vi "ATR.vi"() -> ()   [LabVIEW 2017]
panel:
  out "ArrAHU":string[][](array[string])
  out "ArrEbay":string[][](array[string])
  out "Mort Temp":string[][](array[string])
  out "Aux":string[][](array[string])
  out "Burnin":string[][](array[string])
  out "Temp Algo":string[][](array[string])
  out "Speed":string[][](array[string])
  out "Tempreature calibration":string[][](array[string])
  out "StopTime":string[][](array[string])
  out "Enable":string[][](array[string])
  out "Communication":string[][](array[string])
  out "Visual Inspection":string[][](array[string])
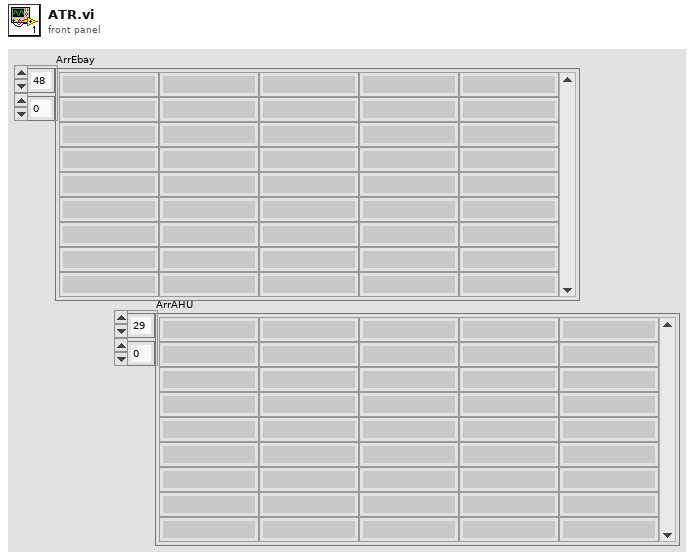
[diagram p1: front panel]
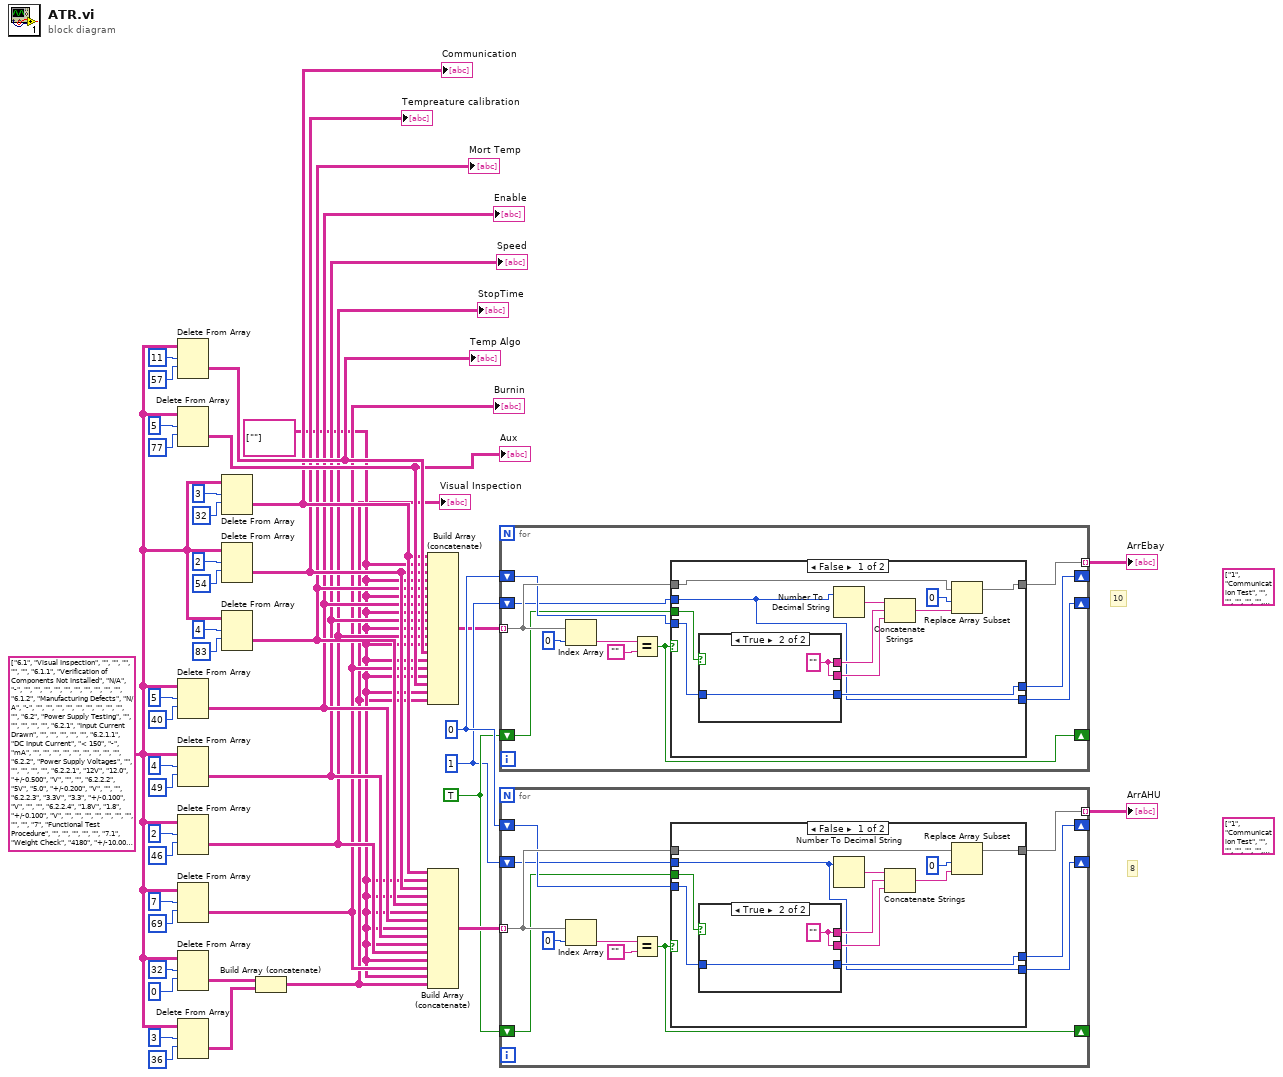
[diagram p0: block diagram]
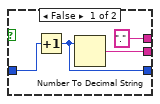
[diagram p2: hidden frame]
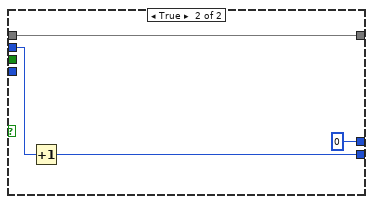
[diagram p3: hidden frame]
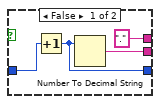
[diagram p4: hidden frame]
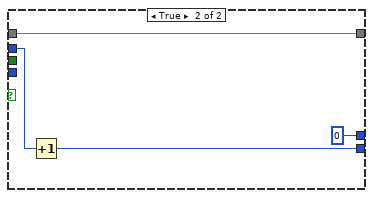
[diagram p5: hidden frame]
diagram:
  (unwired) string[][] [["1", "Communication Test", "", "", "", "", ""], ["1.1", "Serial RS-232", "N/A", "-", "", "", ""], ["1.2", "CAN Bus", "N/A", "-", "", "", ""], ["", "", "", "", "", "", ""], ["2", "Temperature Sensor Calibration Test", "", "", "", "", ""], ["2.1", "Sensor Reading Analog Offset", "0", "+/-0.100", ".", "", ""], ["", "", "", "", "", "", ""], ["3", "Motor Temp. Test", "", "", "", "", ""], ["3.1", "60 Degree", "60", "+/-3.00", "C", "", ""], ["3.2", "90 Degree", "90", "+/-3.00", "C", "", ""], ["3.3", "120 Degree", "120", "+/-3.00", "C", "", ""], ["", "", "", "", "", "", ""], ["4", "Enable Test", "", "", "", "", ""], ["4.1", "Fan Speed at Opened Enable ", "5000", "+/-200.0", "rpm", "", ""], ["4.2", "Fan Speed at Opened Enable ", "0", "+/-200.0", "rpm", "", ""], ["4.3", "Fan Speed at Closed Enable ", "5000", "+/-200.0", "rpm", "", ""], ["4.4", "Motor Rotation Direction", "Counter-clockwise (Inlet)", "-", "", "", ""], ["", "", "", "", "", "", ""], ["5", "Speed Command Test", "", "", "", "", ""], ["5.1", "Fan Speed", "6000", "+/-200.0", "rpm", "", ""], ["5.2", "Fan Speed", "11500", "+/-200.0", "rpm", "", ""], ["5.3", "Fan Speed", "15100", "+/-200.0", "rpm", "", ""], ["", "", "", "", "", "", ""], ["6", "Stop Time Test ", "", "", "", "", ""], ["6.1", "Motor Stop time", "< 50", "-", "sec", "", ""], ["", "", "", "", "", "", ""], ["7", "Burn-in Test", "", "", "", "", ""], ["7.1", "DC Input Current", "50", "+/-5.000", "A", "", ""], ["7.2", "Fan Speed", "15100", "+/-200.0", "rpm", "", ""], ["7.3", "Ambient Temperature", "25", "+/-13.00", "C", "", ""], ["7.4", "After 10 min of operation", "", "-", "C", "", ""], ["7.5", "After 20 min of operation", "", "-", "C", "", ""], ["7.6", "After 30 min of operation", "", "-", "C", "", ""], ["", "", "", "", "", "", ""], ["8", "Visual Inspection", "", "", "", "", ""], ["8.1", "Verification of Components Not Installed", "N/A", "-", "", "", ""], ["", "", "", "", "", "", ""], ["9", "Manufacturing Defects", "N/A", "-", "", "", ""], ["", "", "", "", "", "", ""], ["10", "Power Supply Testing", "", "", "", "", ""], ["10.1", "Input Current Drawn", "", "", "", "", ""], ["10.2", "DC Input Current", "< 150", "-", "mA", "", ""], ["", "", "", "", "", "", ""], ["11", "Power Supply Voltages", "", "", "", "", ""], ["11.1", "12V", "12.0", "+/-0.500", "V", "", ""], ["11.2", "5V", "5.0", "+/-0.200", "V", "", ""], ["11.3", "3.3V", "3.3", "+/-0.100", "V", "", ""], ["11.4", "1.8V", "1.8", "+/-0.100", "V", "", ""], ["", "", "", "", "", "", ""], ["12", "Functional Test Procedure", "", "", "", "", ""], ["12.1", "Weight Check", "4180", "+/-10.00", "gr", "", ""], ["", "", "", "", "", "", ""], ["13", "Insulation Resistance Test", "", "", "", "", ""], ["13.1", "J3.B to Chassis", "> 1M", "-", "W", "", ""], ["13.2", "J1.16 to Chassis", "> 100K", "-", "W", "", ""], ["", "", "", "", "", "", ""], ["14", "Bonding Resistance", "", "", "", "", ""], ["14.1", "J1 Body to Chassis", "< 2m", "-", "W", "", ""], ["14.2", "J2  Body to Chassis", "< 2m", "-", "W", "", ""], ["14.3", "J3  Body to Chassis", "< 2m", "-", "W", "", ""], ["", "", "", "", "", "", ""], ["15", "CANbus Resistance Test", "", "", "", "", ""], ["15.1", "J1.17 to J1.18", "> 10K", "-", "W", "", ""], ["", "", "", "", "", "", ""], ["16", "Sealing Test", "N/A", "-", "", "", ""], ["", "", "", "", "", "", ""], ["17", "Performances Tests", "", "", "", "", ""], ["17.1", "Reverse Polarity Test", "", "", "", "", ""], ["17.2", "DC Input Current", "< 1", "-", "mA", "", ""]] ("ArrAHU 2")
  (unwired) string[][] [["1", "Communication Test", "", "", "", "", ""], ["1.1", "Serial RS-232", "N/A", "-", "", "", ""], ["1.2", "CAN Bus", "N/A", "-", "", "", ""], ["", "", "", "", "", "", ""], ["2", "Temperature Sensor Calibration Test", "", "", "", "", ""], ["2.1", "Sensor Reading Analog Offset", "0", "+/-0.100", ".", "", ""], ["", "", "", "", "", "", ""], ["3", "Motor Temp. Test", "", "", "", "", ""], ["3.1", "60 Degree", "60", "+/-3.00", "C", "", ""], ["3.2", "90 Degree", "90", "+/-3.00", "C", "", ""], ["3.3", "120 Degree", "120", "+/-3.00", "C", "", ""], ["", "", "", "", "", "", ""], ["4", "Enable Test", "", "", "", "", ""], ["4.1", "Fan Speed at Opened Enable ", "5000", "+/-200.0", "rpm", "", ""], ["4.2", "Fan Speed at Opened Enable ", "0", "+/-200.0", "rpm", "", ""], ["4.3", "Fan Speed at Closed Enable ", "5000", "+/-200.0", "rpm", "", ""], ["4.4", "Motor Rotation Direction", "Counter-clockwise (Inlet)", "-", "", "", ""], ["", "", "", "", "", "", ""], ["5", "Speed Command Test", "", "", "", "", ""], ["5.1", "Fan Speed", "6000", "+/-200.0", "rpm", "", ""], ["5.2", "Fan Speed", "11500", "+/-200.0", "rpm", "", ""], ["5.3", "Fan Speed", "15100", "+/-200.0", "rpm", "", ""], ["", "", "", "", "", "", ""], ["6", "Stop Time Test ", "", "", "", "", ""], ["6.1", "Motor Stop time", "< 50", "-", "sec", "", ""], ["", "", "", "", "", "", ""], ["7", "Temperature Control Algorithm Test", "", "", "", "", ""], ["7.1", "Tair <   68 ± 2 oC", "6000", "+/-200.0", "rpm", "", ""], ["7.2", "Measured Temp.", "", "", "C", "", ""], ["7.3", "Tair >= 68 ± 2 oC", "11500", "+/-200.0", "rpm", "", ""], ["7.4", "Transition Temp.", "", "", "C", "", ""], ["7.5", "Tair >= 88 ± 2 oC", "15100", "+/-400.0", "rpm", "", ""], ["7.6", "Transition Temp.", "", "", "C", "", ""], ["7.7", "Tair <= 80 ± 2 oC", "11500", "+/-200.0", "rpm", "", ""], ["7.8", "Transition Temp.", "", "", "C", "", ""], ["7.9", "Tair <= 60 ± 2 oC", "6000", "+/-200.0", "rpm", "", ""], ["7.10", "Transition Temp.", "", "", "C", "", ""], ["", "", "", "", "", "", ""], ["8", "Burn-in Test", "", "", "", "", ""], ["8.1", "DC Input Current", "50", "+/-5.000", "A", "", ""], ["8.2", "Fan Speed", "15100", "+/-200.0", "rpm", "", ""], ["8.3", "Ambient Temperature", "25", "+/-13.00", "C", "", ""], ["8.4", "After 10 min of operation", "", "-", "C", "", ""], ["8.5", "After 20 min of operation", "", "-", "C", "", ""], ["8.6", "After 30 min of operation", "", "-", "C", "", ""], ["", "", "", "", "", "", ""], ["9", "Auxiliary", "", "", "", "", ""], ["9.1", "Auxiliary Cooling Fan ON", "60", "+/-2.00", "C", "", ""], ["9.2", "Fan status", "ON", "-", "-", "", ""], ["9.3", "Auxiliary Cooling Fan OFF", "55", "+/-2.00", "C", "", ""], ["9.4", "Fan status", "OFF", "-", "-", "", ""], ["", "", "", "", "", "", ""], ["10", "Visual Inspection", "", "", "", "", ""], ["10.1", "Verification of Components Not Installed", "N/A", "-", "", "", ""], ["", "", "", "", "", "", ""], ["11", "Manufacturing Defects", "N/A", "-", "", "", ""], ["", "", "", "", "", "", ""], ["12", "Power Supply Testing", "", "", "", "", ""], ["12.1", "Input Current Drawn", "", "", "", "", ""], ["12.2", "DC Input Current", "< 150", "-", "mA", "", ""], ["", "", "", "", "", "", ""], ["13", "Power Supply Voltages", "", "", "", "", ""], ["13.1", "12V", "12.0", "+/-0.500", "V", "", ""], ["13.2", "5V", "5.0", "+/-0.200", "V", "", ""], ["13.3", "3.3V", "3.3", "+/-0.100", "V", "", ""], ["13.4", "1.8V", "1.8", "+/-0.100", "V", "", ""], ["", "", "", "", "", "", ""], ["14", "Functional Test Procedure", "", "", "", "", ""], ["14.1", "Weight Check", "4180", "+/-10.00", "gr", "", ""], ["", "", "", "", "", "", ""], ["15", "Insulation Resistance Test", "", "", "", "", ""], ["15.1", "J3.B to Chassis", "> 1M", "-", "W", "", ""], ["15.2", "J1.16 to Chassis", "> 100K", "-", "W", "", ""], ["", "", "", "", "", "", ""], ["16", "Bonding Resistance", "", "", "", "", ""], ["16.1", "J1 Body to Chassis", "< 2m", "-", "W", "", ""], ["16.2", "J2  Body to Chassis", "< 2m", "-", "W", "", ""], ["16.3", "J3  Body to Chassis", "< 2m", "-", "W", "", ""], ["", "", "", "", "", "", ""], ["17", "CANbus Resistance Test", "", "", "", "", ""], ["17.1", "J1.17 to J1.18", "> 10K", "-", "W", "", ""], ["", "", "", "", "", "", ""], ["18", "Sealing Test", "N/A", "-", "", "", ""], ["", "", "", "", "", "", ""], ["19", "Performances Tests", "", "", "", "", ""], ["19.1", "Reverse Polarity Test", "", "", "", "", ""], ["19.2", "DC Input Current", "< 1", "-", "mA", "", ""]] ("ArrEbay 2")
  w8 = string[][] [[""]] ("array")
  w4 = TRUE
  w3 = 1
  w5 = 0
  w19 = string[][] [["6.1", "Visual Inspection", "", "", "", "", ""], ["6.1.1", "Verification of Components Not Installed", "N/A", "-", "", "", ""], ["", "", "", "", "", "", ""], ["6.1.2", "Manufacturing Defects", "N/A", "-", "", "", ""], ["", "", "", "", "", "", ""], ["6.2", "Power Supply Testing", "", "", "", "", ""], ["6.2.1", "Input Current Drawn", "", "", "", "", ""], ["6.2.1.1", "DC Input Current", "< 150", "-", "mA", "", ""], ["", "", "", "", "", "", ""], ["6.2.2", "Power Supply Voltages", "", "", "", "", ""], ["6.2.2.1", "12V", "12.0", "+/-0.500", "V", "", ""], ["6.2.2.2", "5V", "5.0", "+/-0.200", "V", "", ""], ["6.2.2.3", "3.3V", "3.3", "+/-0.100", "V", "", ""], ["6.2.2.4", "1.8V", "1.8", "+/-0.100", "V", "", ""], ["", "", "", "", "", "", ""], ["7", "Functional Test Procedure", "", "", "", "", ""], ["7.1", "Weight Check", "4180", "+/-10.00", "gr", "", ""], ["", "", "", "", "", "", ""], ["7.2", "Insulation Resistance Test", "", "", "", "", ""], ["7.2.1", "J3.B to Chassis", "> 1M", "-", "W", "", ""], ["7.2.2", "J1.16 to Chassis", "> 100K", "-", "W", "", ""], ["", "", "", "", "", "", ""], ["7.2", "Bonding Resistance", "", "", "", "", ""], ["7.2.3", "J1 Body to Chassis", "< 2m", "-", "W", "", ""], ["7.2.4", "J2  Body to Chassis", "< 2m", "-", "W", "", ""], ["7.2.5", "J3  Body to Chassis", "< 2m", "-", "W", "", ""], ["", "", "", "", "", "", ""], ["7.2.1", "CANbus Resistance Test", "", "", "", "", ""], ["7.2.1.1", "J1.17 to J1.18", "> 10K", "-", "W", "", ""], ["", "", "", "", "", "", ""], ["7.3", "Sealing Test", "N/A", "-", "", "", ""], ["", "", "", "", "", "", ""], ["7.4", "Communication Test", "", "", "", "", ""], ["7.4.1", "Serial RS-232", "N/A", "-", "", "", ""], ["7.4.2", "CAN Bus", "N/A", "-", "", "", ""], ["", "", "", "", "", "", ""], ["7.5", "Performances Tests", "", "", "", "", ""], ["7.5.1", "Reverse Polarity Test", "", "", "", "", ""], ["7.5.1.1", "DC Input Current", "< 1", "-", "mA", "", ""], ["", "", "", "", "", "", ""], ["7.5.2", "Enable Test", "", "", "", "", ""], ["7.5.2.1", "Fan Speed at Opened Enable ", "5000", "+/-200.0", "rpm", "", ""], ["7.5.2.2", "Fan Speed at Opened Enable ", "0", "+/-200.0", "rpm", "", ""], ["7.5.2.3", "Fan Speed at Closed Enable ", "5000", "+/-200.0", "rpm", "", ""], ["7.5.2.4", "Motor Rotation Direction", "Counter-clockwise (Inlet)", "-", "", "", ""], ["", "", "", "", "", "", ""], ["7.5.3", "Stop Time Test ", "", "", "", "", ""], ["7.5.3.1", "Motor Stop time", "< 50", "-", "sec", "", ""], ["", "", "", "", "", "", ""], ["7.5.4", "Speed Command Test", "", "", "", "", ""], ["7.5.4.1", "Fan Speed", "6000", "+/-200.0", "rpm", "", ""], ["7.5.4.2", "Fan Speed", "11500", "+/-200.0", "rpm", "", ""], ["7.5.4.3", "Fan Speed", "15100", "+/-200.0", "rpm", "", ""], ["", "", "", "", "", "", ""], ["7.5.5", "Temperature Sensor Calibration Test", "", "", "", "", ""], ["7.5.5.1", "Sensor Reading Analog Offset", "0", "+/-0.100", ".", "", ""], ["", "", "", "", "", "", ""], ["7.5.6", "Temperature Control Algorithm Test", "", "", "", "", ""], ["7.5.6.1", "Tair <   68 ± 2 oC", "6000", "+/-200.0", "rpm", "", ""], ["7.5.6.2", "Measured Temp.", "", "", "C", "", ""], ["7.5.6.3", "Tair >= 68 ± 2 oC", "11500", "+/-200.0", "rpm", "", ""], ["7.5.6.4", "Transition Temp.", "", "", "C", "", ""], ["7.5.6.5", "Tair >= 88 ± 2 oC", "15100", "+/-400.0", "rpm", "", ""], ["7.5.6.6", "Transition Temp.", "", "", "C", "", ""], ["7.5.6.7", "Tair <= 80 ± 2 oC", "11500", "+/-200.0", "rpm", "", ""], ["7.5.6.8", "Transition Temp.", "", "", "C", "", ""], ["7.5.6.9", "Tair <= 60 ± 2 oC", "6000", "+/-200.0", "rpm", "", ""], ["7.5.6.10", "Transition Temp.", "", "", "C", "", ""], ["", "", "", "", "", "", ""], ["7.5.7", "Burn-in Test", "", "", "", "", ""], ["7.5.7.1", "DC Input Current", "50", "+/-5.000", "A", "", ""], ["7.5.7.2", "Fan Speed", "15100", "+/-200.0", "rpm", "", ""], ["7.5.7.3", "Ambient Temperature", "25", "+/-13.00", "C", "", ""], ["7.5.7.4", "After 10 min of operation", "", "-", "C", "", ""], ["7.5.7.5", "After 20 min of operation", "", "-", "C", "", ""], ["7.5.7.6", "After 30 min of operation", "", "-", "C", "", ""], ["", "", "", "", "", "", ""], ["8", "Auxiliary", "", "", "", "", ""], ["8.1", "Auxiliary Cooling Fan ON", "60", "+/-2.00", "C", "", ""], ["8.2", "Fan status", "ON", "-", "-", "", ""], ["8.3", "Auxiliary Cooling Fan OFF", "55", "+/-2.00", "C", "", ""], ["8.4", "Fan status", "OFF", "-", "-", "", ""], ["", "", "", "", "", "", ""], ["9", "Motor Temp. Test", "", "", "", "", ""], ["9.1", "60 Degree", "60", "+/-3.00", "C", "", ""], ["9.2", "90 Degree", "90", "+/-3.00", "C", "", ""], ["9.3", "120 Degree", "120", "+/-3.00", "C", "", ""]] ("data")
  # "8"
  # "10"
  n1 = Delete From Array(array=w19, length=11, index (row)=57) -> (deleted portion=w18:string[][])  [unwired: 1 in, 1 out]
  "Temp Algo" <- w18
  n2 = Delete From Array(array=w19, length=5, index (row)=77) -> (deleted portion=w17:string[][])  [unwired: 1 in, 1 out]
  "Aux" <- w17
  n3 = Delete From Array(array=w19, length=5, index (row)=40) -> (deleted portion=w12:string[][])  [unwired: 1 in, 1 out]
  "Enable" <- w12
  n4 = Delete From Array(array=w19, length=4, index (row)=49) -> (deleted portion=w11:string[][])  [unwired: 1 in, 1 out]
  "Speed" <- w11
  n5 = Delete From Array(array=w19, length=2, index (row)=46) -> (deleted portion=w10:string[][])  [unwired: 1 in, 1 out]
  "StopTime" <- w10
  n6 = Delete From Array(array=w19, length=7, index (row)=69) -> (deleted portion=w9:string[][])  [unwired: 1 in, 1 out]
  "Burnin" <- w9
  n7 = Delete From Array(array=w19, length=32, index (row)=0) -> (deleted portion=w27:string[][])  [unwired: 1 in, 1 out]
  n8 = Delete From Array(array=w19, length=3, index (row)=36) -> (deleted portion=w26:string[][])  [unwired: 1 in, 1 out]
  n9 = Delete From Array(array=w19, length=3, index (row)=32) -> (deleted portion=w15:string[][])  [unwired: 1 in, 1 out]
  "Communication" <- w15
  n10 = Delete From Array(array=w19, length=2, index (row)=54) -> (deleted portion=w14:string[][])  [unwired: 1 in, 1 out]
  "Tempreature calibration" <- w14
  n11 = Delete From Array(array=w19, length=4, index (row)=83) -> (deleted portion=w13:string[][])  [unwired: 1 in, 1 out]
  "Mort Temp" <- w13
  n12 = Build Array (concatenate)(w27, w26) -> (w2:string[][])
  "Visual Inspection" <- w2
  n13 = Build Array (concatenate)(w15, w8, w14, w8, w13, w8, w12, w8, w11, w8, w10, w8, w18, w8, w9, w8, w17, w8, w2) -> (w1:string[][])
  n14 = Build Array (concatenate)(w15, w8, w14, w8, w13, w8, w12, w8, w11, w8, w10, w8, w9, w8, w2) -> (w7:string[][])
  n15 = for {
    tunnel: w1 -> [w53] mode=indexing
    tunnel: [w54] -> w16 mode=indexing
    shift-right: [w48] -> _
    shift-left: w5 -> [w49]
    shift-right: [w46] -> _
    shift-left: w3 -> [w47]
    shift-right: [w45] -> _
    shift-left: w4 -> [w44]
    n16 = Index Array(array=w53, index=0) -> (element=w51:string)
    n17 = Equal?(x=w51, y="") -> (x = y?=w45:bool)
    n18 = case shown="False" w45 {
      tunnel: w49 -> [w59 _]
      tunnel: [w62 w75] -> w54
      tunnel: w53 -> [w61 w75]
      tunnel: [w60 0] -> w48
      tunnel: w47 -> [w56 w74]
      tunnel: [w56 w73] -> w46
      tunnel: w44 -> [w55 _]
      frame False {
        n19 = case shown="True" w55 {
          tunnel: [w69 w71] -> w64
          tunnel: [w68 w70] -> w60
          tunnel: w59 -> [w67 w70]
          tunnel: ["." ("string") w71] -> w57
          frame False {
            n20 = Increment(x=w67) -> (x+1=w68:i32)
            n21 = Number To Decimal String(number=w68) -> (decimal integer string=w69:string)  [unwired: 1 in]
          }
          frame True {
            w71 = "" ("string")
          }
        }
        n22 = Number To Decimal String(number=w56) -> (decimal integer string=w58:string)  [unwired: 1 in]
        n23 = Concatenate Strings(w58, w57, w64) -> (w63:string)
        n24 = Replace Array Subset(array=w61, new element=w63, index=0) -> (w62:string[])
      }
      frame True {
        n25 = Increment(x=w74) -> (x+1=w73:i32)
      }
    }
  }
  "ArrEbay" <- w16
  n26 = for {
    tunnel: w7 -> [w85] mode=indexing
    tunnel: [w86] -> w6 mode=indexing
    shift-right: [w80] -> _
    shift-left: w5 -> [w81]
    shift-right: [w78] -> _
    shift-left: w3 -> [w79]
    shift-right: [w77] -> _
    shift-left: w4 -> [w76]
    n27 = Index Array(array=w85, index=0) -> (element=w83:string)
    n28 = Equal?(x=w83, y="") -> (x = y?=w77:bool)
    n29 = case shown="False" w77 {
      tunnel: w81 -> [w91 _]
      tunnel: [w94 w107] -> w86
      tunnel: w85 -> [w93 w107]
      tunnel: [w92 0] -> w80
      tunnel: w79 -> [w88 w106]
      tunnel: [w88 w105] -> w78
      tunnel: w76 -> [w87 _]
      frame False {
        n30 = case shown="True" w87 {
          tunnel: [w101 w103] -> w96
          tunnel: [w100 w102] -> w92
          tunnel: w91 -> [w99 w102]
          tunnel: ["." ("string") w103] -> w89
          frame False {
            n31 = Increment(x=w99) -> (x+1=w100:i32)
            n32 = Number To Decimal String(number=w100) -> (decimal integer string=w101:string)  [unwired: 1 in]
          }
          frame True {
            w103 = "" ("string")
          }
        }
        n33 = Number To Decimal String(number=w88) -> (decimal integer string=w90:string)  [unwired: 1 in]
        n34 = Concatenate Strings(w90, w89, w96) -> (w95:string)
        n35 = Replace Array Subset(array=w93, new element=w95, index=0) -> (w94:string[])
      }
      frame True {
        n36 = Increment(x=w106) -> (x+1=w105:i32)
      }
    }
  }
  "ArrAHU" <- w6
